vi "Update Stations.vi"(8 "error in (no error)":errorcluster, 10 "Combo Value":string, 11 "OPC Server in":refnum<class "PLC Sim Controller Actor.lvclass">) -> (0 "error out":errorcluster, 3 "OPC Server out":refnum<class "PLC Sim Controller Actor.lvclass">)   [LabVIEW 2019, in "PLC Sim Controller Actor.lvlib" / "PLC Sim Controller Actor.lvclass"]
uses:
  PLC Sim Controller Actor.lvclass
  PLC Sim Controller Actor.lvclass/PLC Sim Controller Actor.ctl
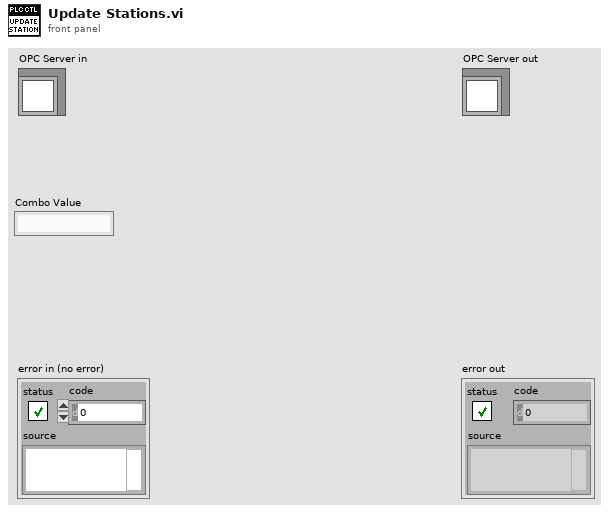
[diagram p1: front panel]
types:
  T1 = map{string, refnum<class "Message Enqueuer.lvclass">}
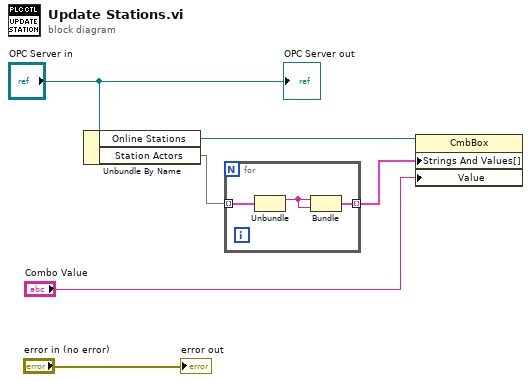
[diagram p0: block diagram]
diagram:
  n1 = Unbundle By Name("OPC Server in") -> ("Online Stations"=w5:refnum<vi>, "Station Actors"=w4:T1)
  n2 = for {
    tunnel: w4 -> [w9] mode=indexing
    tunnel: [w7] -> w3 mode=indexing
    n3 = Unbundle(w9) -> (w8:string)  [unwired: 1 out]
    n4 = Bundle(w8, w8) -> (w7:cluster{string, string})  [unwired: 1 in]
  }
  n5 = property class="CmbBox"(reference=w5, "Strings And Values[]"=w3, "Value"="Combo Value") -> ()  [unwired: 1 in, 2 out]
  "error out" <- "error in (no error)"
  "OPC Server out" <- "OPC Server in"
